vi "Send Email.vi"(8 "error in (no error)":errorcluster, 11 "StmpEmail in":refnum<class "StmpEmail.lvclass">) -> (0 "error out":errorcluster, 3 "StmpEmail out":refnum<class "StmpEmail.lvclass">)   [LabVIEW 2015, in "StmpEmail.lvclass"]
uses:
  StmpEmail.lvclass
  StmpEmail.lvclass/StmpEmail.ctl
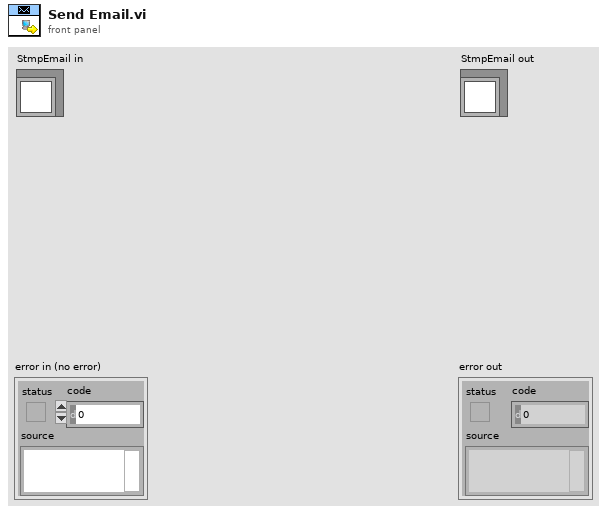
[diagram p1: front panel]
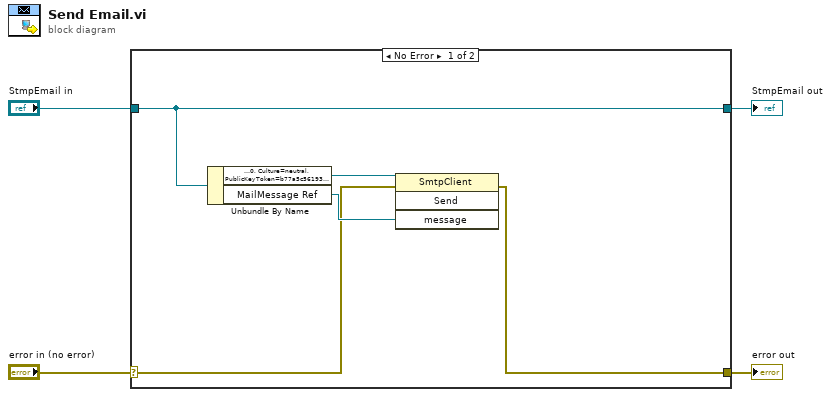
[diagram p0: block diagram]
diagram:
  n1 = case shown="No Error" "error in (no error)" {
    selector: "error in (no error)" -> [w6 w11]
    tunnel: [w5 w11] -> w3
    tunnel: [w9 w10] -> w1
    tunnel: "StmpEmail in" -> [w9 w10]
    frame No Error {
      n2 = Unbundle By Name(w9) -> ("SmtpEamil Ref"=w8:refnum<k24>, "MailMessage Ref"=w7:refnum<k24>)
      n3 = invoke class="SmtpClient" method="Send"(reference=w8, error in=w6, "message"=w7) -> (error out=w5:errorcluster)  [unwired: 1 in, 3 out]
    }
    frame Error {
    }
  }
  "error out" <- w3
  "StmpEmail out" <- w1
